vi "Establish Mapped Drive Conn.vi"(11 "Data Logging Directory IN":path) -> ()   [LabVIEW 2018]
panel:
  out "TestData Error":errorcluster
  out "Drive Reconnect Message":string
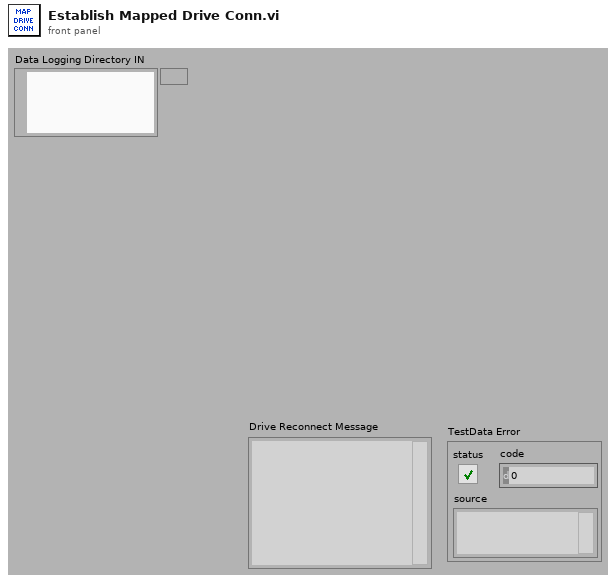
[diagram p1: front panel]
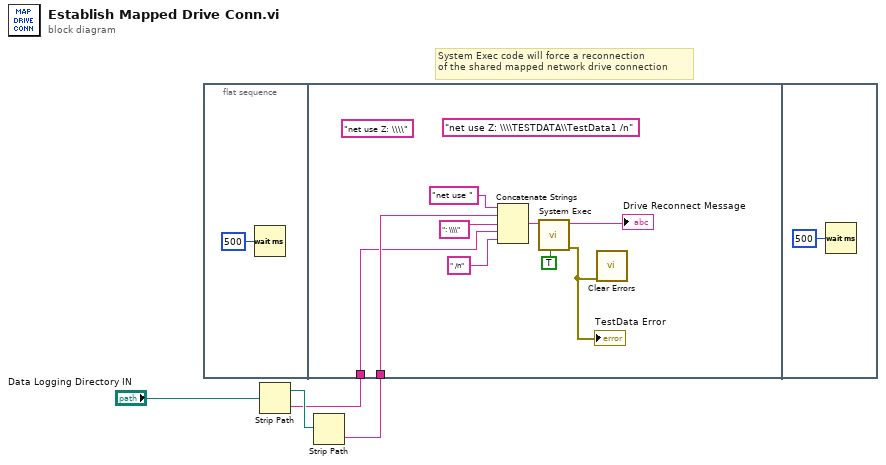
[diagram p0: block diagram]
diagram:
  # "System Exec code will force a reconnection\nof the shared mapped network drive connection"
  n1 = flat-sequence {
    tunnel: w2 -> [w9]
    tunnel: w1 -> [w7]
    frame #0 {
      n2 = Wait (ms)(milliseconds to wait=u32 500) -> ()  [unwired: 1 out]
    }
    frame #1 {
      (unwired) "net use Z: \\\\"
      (unwired) "net use Z: \\\\TESTDATA\\TestData1 /n"
      n3 = Concatenate Strings("net use ", w9, ": \\\\", w7, " /n") -> (w11:string)
      n4 = call <vilib>:"System Exec.vi"("run minimized? (F)"=TRUE, "command line"=w11) -> ("error out"=w12:errorcluster, "standard output"=→"Drive Reconnect Message":string)  [unwired: 6 in, 2 out]
      "TestData Error" <- w12
      n5 = call <vilib>:"Clear Errors.vi"("error in (no error)"=w12) -> ()  [unwired: 5 in, 2 out]
    }
    frame #2 {
      n6 = Wait (ms)(milliseconds to wait=u32 500) -> ()  [unwired: 1 out]
    }
  }
  n7 = Strip Path(path="Data Logging Directory IN") -> (stripped path=w3:path, name=w1:string)
  n8 = Strip Path(path=w3) -> (name=w2:string)  [unwired: 1 out]
